vi "Get Transfer UIs.vi"(8 "error in (no error)":errorcluster, 11 "Component UI in":refnum<class "Default Buffer Converter User Interfaces.lvclass">) -> (0 "error out":errorcluster, 1 "Tx Transfer UI":refnum<class "User Interface.lvclass">, 2 "Rx Transfer UI":refnum<class "User Interface.lvclass">, 3 "Component UI out":refnum<class "Default Buffer Converter User Interfaces.lvclass">)   [LabVIEW 2017, in "DSF Core.lvlib" / "Default Buffer Converter User Interfaces.lvclass"]
uses:
  Default Buffer Converter User Interfaces.lvclass
  Classes/User Interface/User Interface.lvclass
  Transfer/Default Buffer Converter Transfers UI.lvclass
  C:/Git/DSF/Core/Classes/User Interface/User Interface.lvclass
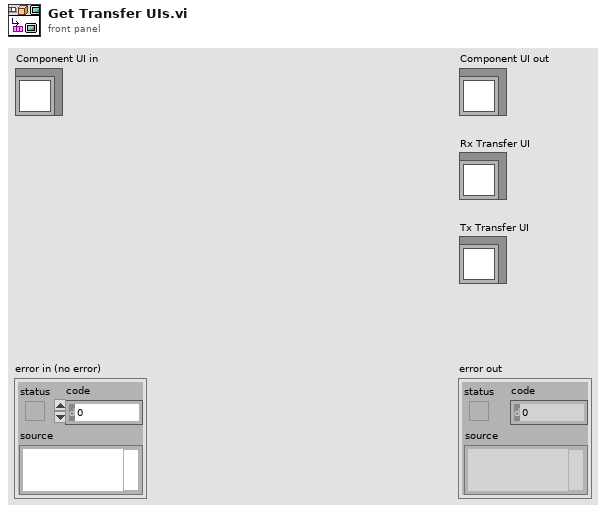
[diagram p1: front panel]
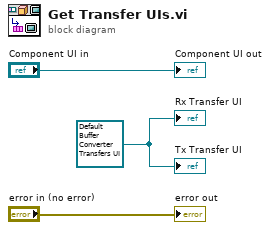
[diagram p0: block diagram]
diagram:
  w1 = refnum<class "Default Buffer Converter Transfers UI.lvclass"> refnum ("DSF Core.lvlib:DSF Buffer Converter Transfers UI.lvclass")
  "error out" <- "error in (no error)"
  "Component UI out" <- "Component UI in"
  "Rx Transfer UI" <- w1
  "Tx Transfer UI" <- w1
